vi "Ejercicio 5 Acabado.vi"() -> ()   [LabVIEW 2021]
panel:
  out "appended array":bool[](array[boolean])
  out "x > y?":bool
  in  "stop 3":bool
  in  "stop 2":bool
  in  "stop":bool
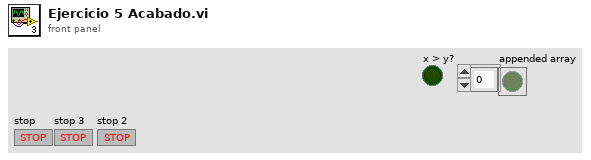
[diagram p1: front panel]
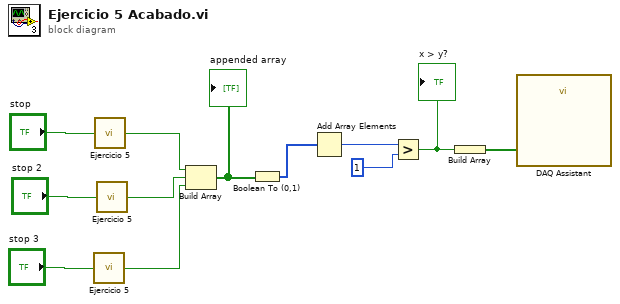
[diagram p0: block diagram]
diagram:
  n1 = call "Ejercicio 5.vi"("stop"="stop 3") -> ("x > y?"=w7:bool)
  n2 = call "Ejercicio 5.vi"("stop"="stop") -> ("x > y?"=w9:bool)
  n3 = call "Ejercicio 5.vi"("stop"="stop 2") -> ("x > y?"=w8:bool)
  n4 = Build Array(w9, w8, w7) -> (w5:bool[])
  "appended array" <- w5
  n5 = Boolean To (0,1)(Boolean=w5) -> (0, 1=w6:i16[])
  n6 = Add Array Elements(numeric array=w6) -> (sum=w4:i16)
  n7 = Greater?(x=w4, y=1) -> (0:w2:bool)
  "x > y?" <- w2
  n8 = Build Array(w2) -> (w1:bool[])
  n9 = call "DAQ Assistant"("data"=w1) -> ()  [unwired: 17 in, 2 out]
